vi "开机添加默认配置文件.vi"(8 "error in (no error)":errorcluster caption="错误输入（无错误）", 11 "恢复默认方式":enum16{"无配置开机恢复", "手动恢复"}(ring)) -> (0 "error out":errorcluster caption="错误输出")   [LabVIEW 2016, in "环境动力监测库.lvlib"]
uses:
  <vilib>/Utility/config.llb/NI_LVConfig.lvlib
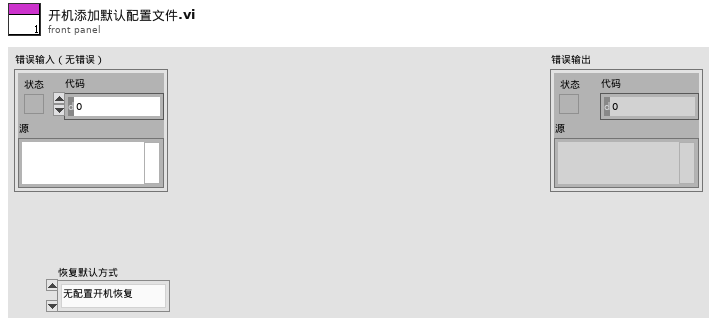
[diagram p1: front panel]
types:
  T1 = cluster{"监测项描述:输出":string, "端口":enum16{"AI0", "AI1", "AI2", "AI3", "AI4", "DI0", "DI1", "DI2", "DI3", "DI4", "DI5", "DI6", "DI7", "DO0", "DO1", "DO2", "DO3", "DO4", "DO5", "DO6", "DO7", "X0", "X1", "X2", "X3", "X4", "X5", "X6", "X7", "X8", "X9", "X10", "X11", "X12", "X13", "X14", "X15", "X16", "X17", "X18", "X19", "X20", "X21", "X22", "X23"}, "告警方式":enum32{"禁用告警", "闭合告警", "断开告警"}, "传感器型号":enum16{"PLC", "ZLAN", "ART"}, "声光告警启用":bool}
  T2 = typedef "NI_LVConfig.lvlib/Config Data RefNum.ctl" = refnum<k1>
  T3 = cluster{"监测项描述:输出":string, "连接方式":enum16{"串口", "TCP"}, "端口":string, "IP address:":string, "Port:":string, "站号":u64, "传感器型号":string, "波特率":u64, "data bits":u64, "停止位":u16, "奇偶校验":u16}
  T4 = cluster{"监测项描述:输出":string, "端口":enum16{"AI0", "AI1", "AI2", "AI3", "AI4", "DI0", "DI1", "DI2", "DI3", "DI4", "DO0", "DO1", "DO2", "DO3", "DO4", "X0", "X1", "X2", "X3", "X4", "X5", "X6", "X7", "X8", "X9"}, "告警方式":enum32{"禁用告警", "闭合告警", "断开告警"}, "传感器型号":enum16{"PLC", "ZLAN"}}
  T5 = enum16{"AI0", "AI1", "AI2", "AI3", "AI4", "DI0", "DI1", "DI2", "DI3", "DI4", "DI5", "DI6", "DI7", "DO0", "DO1", "DO2", "DO3", "DO4", "DO5", "DO6", "DO7", "X0", "X1", "X2", "X3", "X4", "X5", "X6", "X7", "X8", "X9"}[]
  T6 = cluster{"漏水监测配置":cluster{"监测项描述:输出":string, "端口:":enum16{"AI0", "AI1", "AI2", "AI3", "AI4", "DI0", "DI1", "DI2", "DI3", "DI4", "DI5", "DI6", "DI7", "DO0", "DO1", "DO2", "DO3", "DO4", "DO5", "DO6", "DO7", "X0", "X1", "X2", "X3", "X4", "X5", "X6", "X7", "X8", "X9", "X10", "X11", "X12", "X13", "X14", "X15", "X16", "X17", "X18", "X19", "X20", "X21", "X22", "X23"}, "告警参数:":enum32{"禁用告警", "闭合告警", "断开告警"}, "传感器型号:":enum16{"PLC", "ZLAN", "ART"}, "声光告警启用":bool}, "门禁开关监测配置":cluster{"监测项描述:输出":string, "端口:":enum16{"AI0", "AI1", "AI2", "AI3", "AI4", "DI0", "DI1", "DI2", "DI3", "DI4", "DI5", "DI6", "DI7", "DO0", "DO1", "DO2", "DO3", "DO4", "DO5", "DO6", "DO7", "X0", "X1", "X2", "X3", "X4", "X5", "X6", "X7", "X8", "X9", "X10", "X11", "X12", "X13", "X14", "X15", "X16", "X17", "X18", "X19", "X20", "X21", "X22", "X23"}, "告警参数:":enum32{"禁用告警", "闭合告警", "断开告警"}, "传感器型号:":enum16{"PLC", "ZLAN", "ART"}, "声光告警启用":bool}, "门禁开关监测配置2":cluster{"监测项描述:输出":string, "端口:":enum16{"AI0", "AI1", "AI2", "AI3", "AI4", "DI0", "DI1", "DI2", "DI3", "DI4", "DI5", "DI6", "DI7", "DO0", "DO1", "DO2", "DO3", "DO4", "DO5", "DO6", "DO7", "X0", "X1", "X2", "X3", "X4", "X5", "X6", "X7", "X8", "X9", "X10", "X11", "X12", "X13", "X14", "X15", "X16", "X17", "X18", "X19", "X20", "X21", "X22", "X23"}, "告警参数:":enum32{"禁用告警", "闭合告警", "断开告警"}, "传感器型号:":enum16{"PLC", "ZLAN", "ART"}, "声光告警启用":bool}, "温湿度监测配置":cluster{"监测项描述:输出":string, "端口:":enum16{"AI0", "AI1", "AI2", "AI3", "AI4", "DI0", "DI1", "DI2", "DI3", "DI4", "DI5", "DI6", "DI7", "DO0", "DO1", "DO2", "DO3", "DO4", "DO5", "DO6", "DO7", "X0", "X1", "X2", "X3", "X4", "X5", "X6", "X7", "X8", "X9", "X10", "X11", "X12", "X13", "X14", "X15", "X16", "X17", "X18", "X19", "X20", "X21", "X22", "X23"}, "告警参数:":enum32{"禁用告警", "闭合告警", "断开告警"}, "传感器型号:":enum16{"PLC", "ZLAN", "ART"}, "声光告警启用":bool}, "烟雾监测配置":cluster{"监测项描述:输出":string, "端口:":enum16{"AI0", "AI1", "AI2", "AI3", "AI4", "DI0", "DI1", "DI2", "DI3", "DI4", "DI5", "DI6", "DI7", "DO0", "DO1", "DO2", "DO3", "DO4", "DO5", "DO6", "DO7", "X0", "X1", "X2", "X3", "X4", "X5", "X6", "X7", "X8", "X9", "X10", "X11", "X12", "X13", "X14", "X15", "X16", "X17", "X18", "X19", "X20", "X21", "X22", "X23"}, "告警参数:":enum32{"禁用告警", "闭合告警", "断开告警"}, "传感器型号:":enum16{"PLC", "ZLAN", "ART"}, "声光告警启用":bool}, "冰箱监测配置":cluster{"监测项描述:输出":string, "端口:":enum16{"AI0", "AI1", "AI2", "AI3", "AI4", "DI0", "DI1", "DI2", "DI3", "DI4", "DI5", "DI6", "DI7", "DO0", "DO1", "DO2", "DO3", "DO4", "DO5", "DO6", "DO7", "X0", "X1", "X2", "X3", "X4", "X5", "X6", "X7", "X8", "X9", "X10", "X11", "X12", "X13", "X14", "X15", "X16", "X17", "X18", "X19", "X20", "X21", "X22", "X23"}, "告警参数:":enum32{"禁用告警", "闭合告警", "断开告警"}, "传感器型号:":enum16{"PLC", "ZLAN", "ART"}, "声光告警启用":bool}, "排气扇监测配置":cluster{"监测项描述:输出":string, "端口:":enum16{"AI0", "AI1", "AI2", "AI3", "AI4", "DI0", "DI1", "DI2", "DI3", "DI4", "DI5", "DI6", "DI7", "DO0", "DO1", "DO2", "DO3", "DO4", "DO5", "DO6", "DO7", "X0", "X1", "X2", "X3", "X4", "X5", "X6", "X7", "X8", "X9", "X10", "X11", "X12", "X13", "X14", "X15", "X16", "X17", "X18", "X19", "X20", "X21", "X22", "X23"}, "告警参数:":enum32{"禁用告警", "闭合告警", "断开告警"}, "传感器型号:":enum16{"PLC", "ZLAN", "ART"}, "声光告警启用":bool}, "红外入侵监测配置":cluster{"监测项描述:输出":string, "端口:":enum16{"AI0", "AI1", "AI2", "AI3", "AI4", "DI0", "DI1", "DI2", "DI3", "DI4", "DI5", "DI6", "DI7", "DO0", "DO1", "DO2", "DO3", "DO4", "DO5", "DO6", "DO7", "X0", "X1", "X2", "X3", "X4", "X5", "X6", "X7", "X8", "X9", "X10", "X11", "X12", "X13", "X14", "X15", "X16", "X17", "X18", "X19", "X20", "X21", "X22", "X23"}, "告警参数:":enum32{"禁用告警", "闭合告警", "断开告警"}, "传感器型号:":enum16{"PLC", "ZLAN", "ART"}, "声光告警启用":bool}, "振动监测配置":cluster{"监测项描述:输出":string, "端口:":enum16{"AI0", "AI1", "AI2", "AI3", "AI4", "DI0", "DI1", "DI2", "DI3", "DI4", "DI5", "DI6", "DI7", "DO0", "DO1", "DO2", "DO3", "DO4", "DO5", "DO6", "DO7", "X0", "X1", "X2", "X3", "X4", "X5", "X6", "X7", "X8", "X9", "X10", "X11", "X12", "X13", "X14", "X15", "X16", "X17", "X18", "X19", "X20", "X21", "X22", "X23"}, "告警参数:":enum32{"禁用告警", "闭合告警", "断开告警"}, "传感器型号:":enum16{"PLC", "ZLAN", "ART"}, "声光告警启用":bool}, "废液监测配置":cluster{"监测项描述:输出":string, "端口:":enum16{"AI0", "AI1", "AI2", "AI3", "AI4", "DI0", "DI1", "DI2", "DI3", "DI4", "DI5", "DI6", "DI7", "DO0", "DO1", "DO2", "DO3", "DO4", "DO5", "DO6", "DO7", "X0", "X1", "X2", "X3", "X4", "X5", "X6", "X7", "X8", "X9", "X10", "X11", "X12", "X13", "X14", "X15", "X16", "X17", "X18", "X19", "X20", "X21", "X22", "X23"}, "告警参数:":enum32{"禁用告警", "闭合告警", "断开告警"}, "传感器型号:":enum16{"PLC", "ZLAN", "ART"}, "声光告警启用":bool}, "废液监测配置2":cluster{"监测项描述:输出":string, "端口:":enum16{"AI0", "AI1", "AI2", "AI3", "AI4", "DI0", "DI1", "DI2", "DI3", "DI4", "DI5", "DI6", "DI7", "DO0", "DO1", "DO2", "DO3", "DO4", "DO5", "DO6", "DO7", "X0", "X1", "X2", "X3", "X4", "X5", "X6", "X7", "X8", "X9", "X10", "X11", "X12", "X13", "X14", "X15", "X16", "X17", "X18", "X19", "X20", "X21", "X22", "X23"}, "告警参数:":enum32{"禁用告警", "闭合告警", "断开告警"}, "传感器型号:":enum16{"PLC", "ZLAN", "ART"}, "声光告警启用":bool}}
  T7 = cluster{"市电监测":bool, "用水量监测":bool, "烟雾监测":bool, "温度湿度":bool, "振动监测":bool, "红外入侵监测":bool, "漏水监测":bool, "门禁开关监测":bool, "门禁开关监测2":bool, "视频监测":bool, "UPS监测":bool, "空调监测":bool, "冰箱监测":bool, "排气扇监测":bool, "蓄电池监测":bool, "蓄电池监测2":bool, "GPS监测":bool, "北斗监测":bool, "气象监测":bool, "智能门禁监测":bool, "废液监测":bool, "废液监测2":bool}
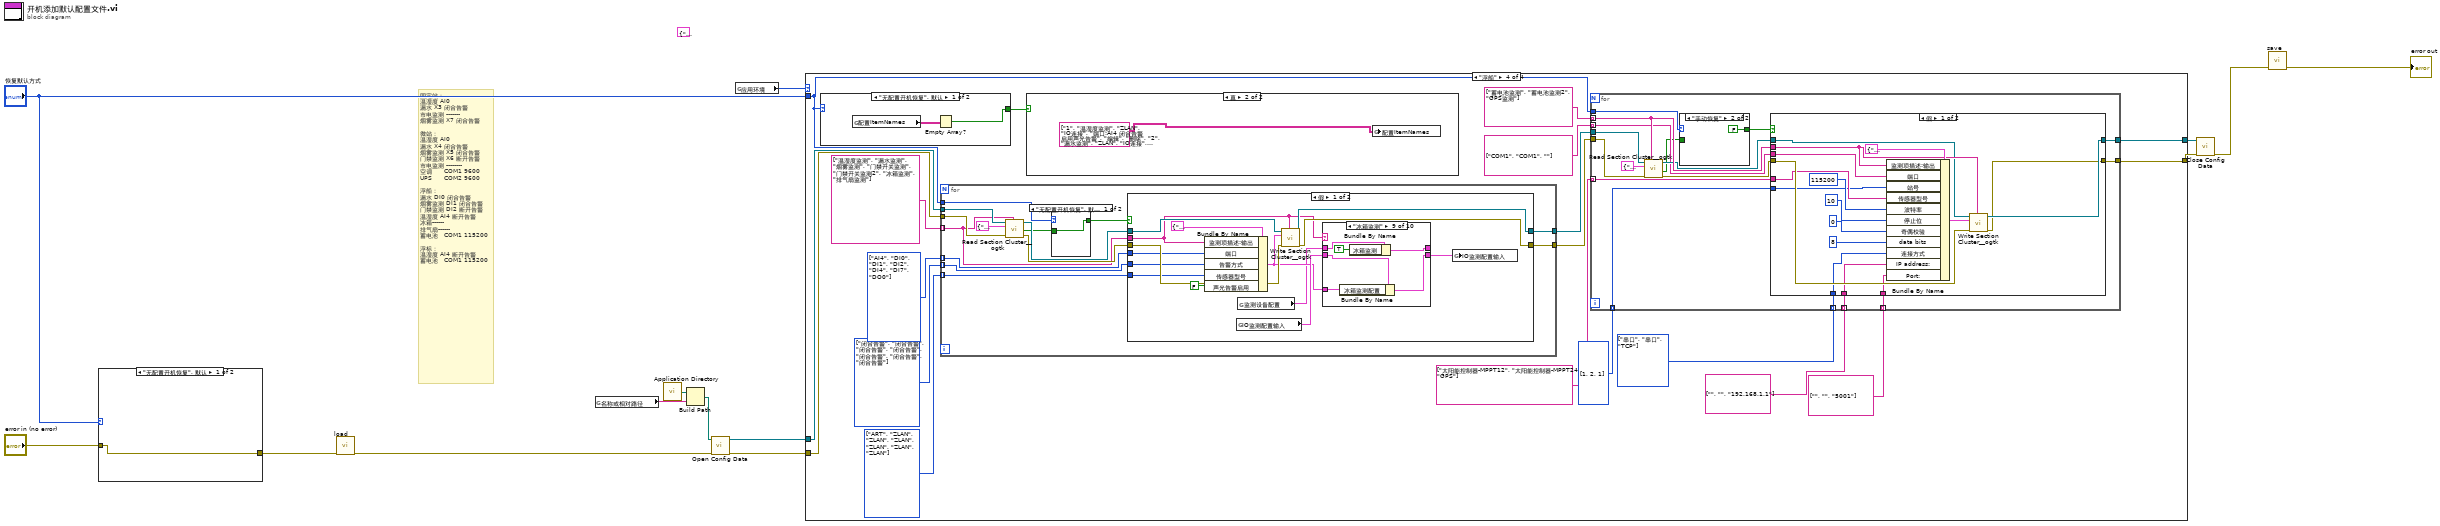
[diagram p0: block diagram]
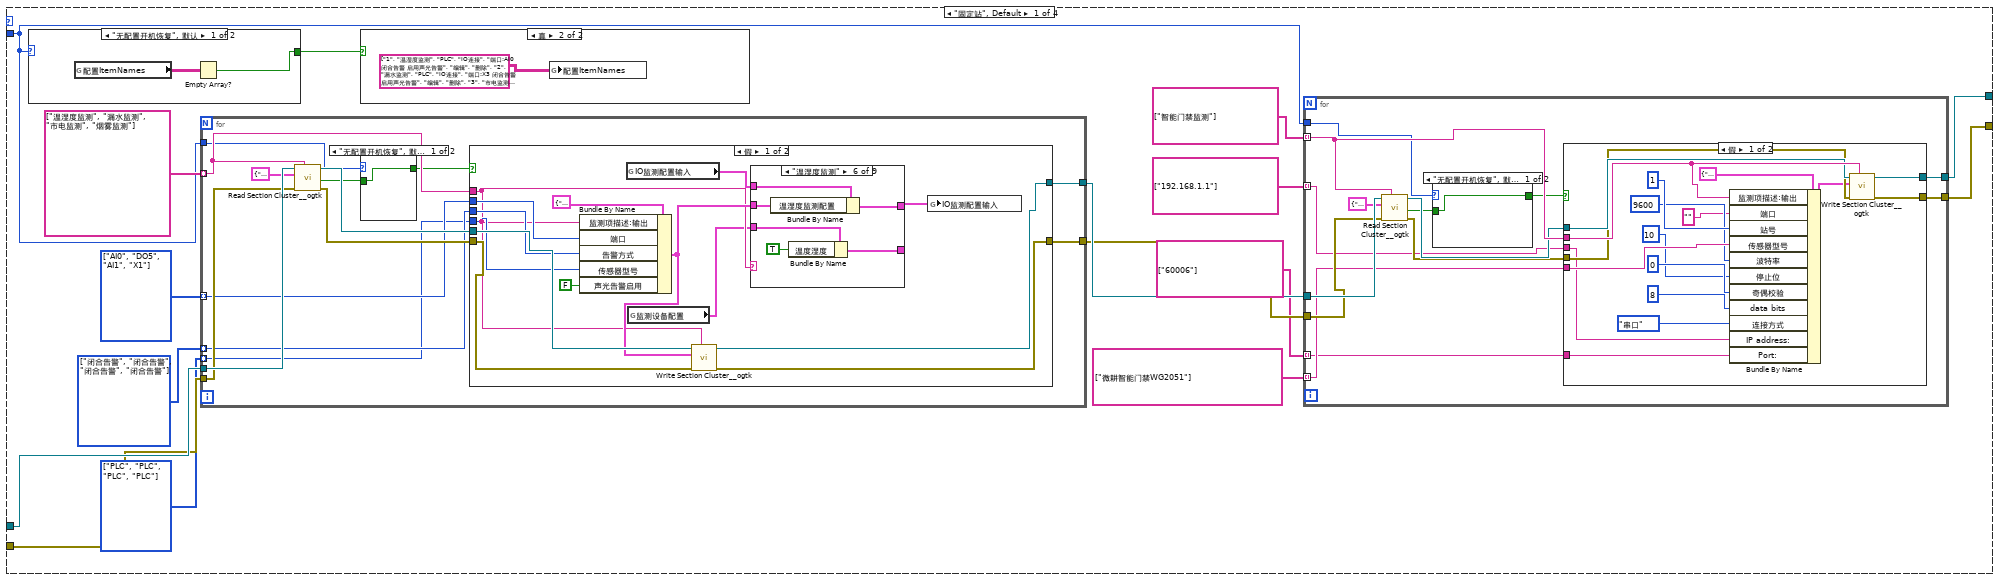
[diagram p3: hidden frame]
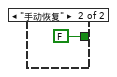
[diagram p4: hidden frame]
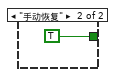
[diagram p6: hidden frame]
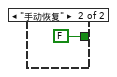
[diagram p8: hidden frame]
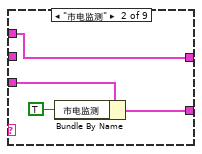
[diagram p10: hidden frame]
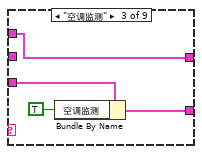
[diagram p11: hidden frame]
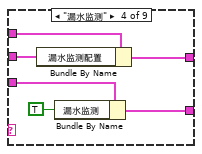
[diagram p12: hidden frame]
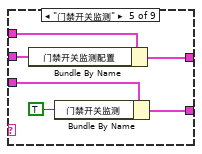
[diagram p13: hidden frame]
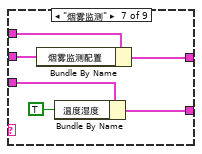
[diagram p14: hidden frame]
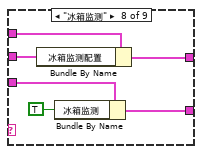
[diagram p15: hidden frame]
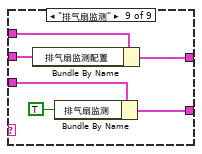
[diagram p16: hidden frame]
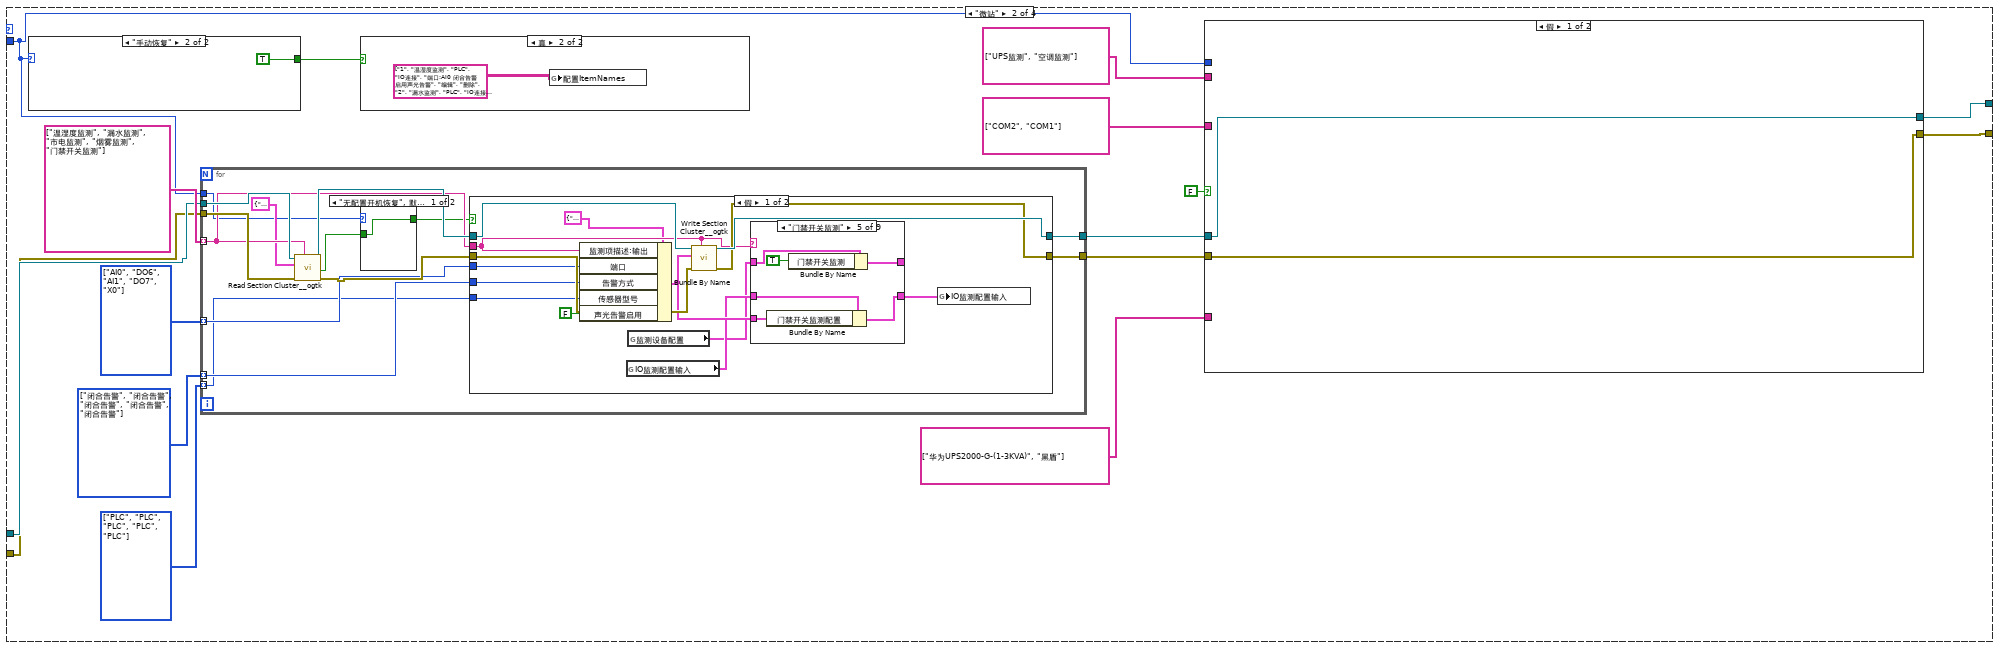
[diagram p18: hidden frame]
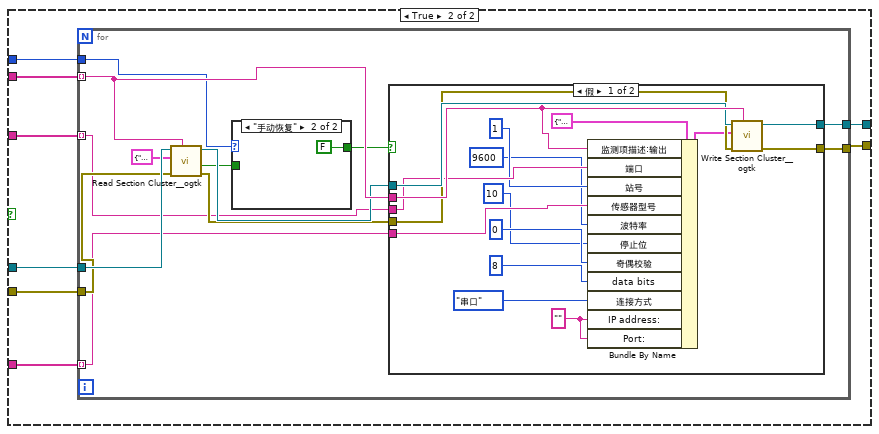
[diagram p19: hidden frame]
diagram:
  (unwired) T1 {"监测项描述:输出"="", "端口"=enum."AI0", "告警方式"=enum."禁用告警", "传感器型号"=enum."PLC", "声光告警启用"=FALSE} ("簇1输入")
  # "固定站：\n温湿度 AI0\n漏水 X3 闭合告警\n市电监测 -------\n烟雾监测 X7 闭合告警\n\n微站：\n温湿度 AI0\n漏水 X4 闭合告警\n烟雾监测 X5 闭合告警\n门禁监测 X6 断开告警\n市电监测 --------\n空调      COM1 9600\nUPS      COM2 9600\n\n浮船：\n漏水 DI0 闭合告警\n烟雾监测 DI1 闭合告警\n门禁监测 DI2 断开告警\n温湿度 AI4 断开告警\n冰箱------\n排气扇------\n蓄电池   COM1 115200\n\n浮标：\n温湿度 AI4 断开告警\n蓄电池   COM1 115200"
  n1 = case shown="\"无配置开机恢复\", 默认" "恢复默认方式" {
    tunnel: "error in (no error)" -> [w15 w16]
    tunnel: [w15 w16] -> w3
    frame "无配置开机恢复", Default {
    }
    frame "手动恢复" {
    }
  }
  n2 = call "load.vi"("error in (no error)"=w3) -> ("error out"=w7:errorcluster)  [unwired: 10 in]
  n3 = global read "内部交互全局变量.vi" "名称或相对路径"() -> (w4:string)
  n4 = call <vilib>:"Application Directory.vi"() -> ("Application Directory"=w13:path)
  n5 = Build Path(base path=w13, name or relative path=w4) -> (appended path=w12:path)
  n6 = call <vilib>:"Open Config Data.vi"("error in (no error)"=w7, "configuration file path"=w12) -> ("error out"=w10:errorcluster, "refnum"=w11:T2)  [unwired: 7 in, 1 out]
  n7 = global read "外部交互全局变量.vi" "应用环境"() -> (w14:enum16{"固定站", "微站", "浮标", "浮船"})
  n8 = case shown="\"浮船\"" w14 {
    tunnel: w11 -> [w31 w164 w304 w438]
    tunnel: w10 -> [w30 w163 w303 w437]
    tunnel: [w19 w159 w299 w433] -> w9
    tunnel: [w18 w158 w298 w432] -> w8
    tunnel: "恢复默认方式" -> [w20 w151 w291 w425]
    frame "固定站", Default {
      w27 = enum16{"PLC", "ZLAN"}[] [enum."PLC", enum."PLC", enum."PLC", enum."PLC"] items=["PLC", "ZLAN"]
      w28 = enum32{"禁用告警", "闭合告警", "断开告警"}[] [enum."闭合告警", enum."闭合告警", enum."闭合告警", enum."闭合告警"] items=["禁用告警", "闭合告警", "断开告警"]
      w29 = T5 [enum."AI0", enum."DO5", enum."AI1", enum."X1"] items=["AI0", "AI1", "AI2", "AI3", "AI4", "DI0", "DI1", "DI2", "DI3", "DI4", "DI5", "DI6", "DI7", "DO0", "DO1", "DO2", "DO3", "DO4", "DO5", "DO6", "DO7", "X0", "X1", "X2", "X3", "X4", "X5", "X6", "X7", "X8", "X9"]
      n9 = case shown="\"无配置开机恢复\", 默认" w20 {
        tunnel: [w68 TRUE ("empty?")] -> w26
        frame "无配置开机恢复", Default {
          n10 = global read "断电保存全局变量.vi" "配置ItemNames"() -> (w69:string[][])
          n11 = Empty Array?(array=w69) -> (empty?=w68:bool)
        }
        frame "手动恢复" {
        }
      }
      n12 = for {
        tunnel: string[] ["温湿度监测", "漏水监测", "市电监测", "烟雾监测"] -> [w81] mode=indexing
        tunnel: w31 -> [w85]
        tunnel: w30 -> [w84]
        tunnel: w29 -> [w80] mode=indexing
        tunnel: w28 -> [w79] mode=indexing
        tunnel: w27 -> [w78] mode=indexing
        tunnel: [w77] -> w22
        tunnel: [w76] -> w21
        tunnel: w20 -> [w72]
        n13 = call <userlib>:"Read Section Cluster__ogtk.vi"("section (optional)"=w81, "error in (no error)"=w84, "Section Formatted Cluster Type"=T4 {"监测项描述:输出"="烟雾监测", "端口"=enum."X8", "告警方式"=enum."闭合告警", "传感器型号"=enum."PLC"} ("簇1输入"), "refnum"=w85) -> ("error out"=w82:errorcluster, "all found?"=w74:bool, "dup refnum"=w83:T2)  [unwired: 3 in, 2 out]
        n14 = case shown="\"无配置开机恢复\", 默认" w72 {
          tunnel: [w86 FALSE] -> w73
          tunnel: w74 -> [w86 _]
          frame "无配置开机恢复", Default {
          }
          frame "手动恢复" {
          }
        }
        n15 = case shown="假" w73 {
          tunnel: w83 -> [w101 w149]
          tunnel: w82 -> [w100 w148]
          tunnel: w81 -> [w92 _]
          tunnel: w80 -> [w99 _]
          tunnel: w79 -> [w94 _]
          tunnel: w78 -> [w98 _]
          tunnel: [w97 w149] -> w77
          tunnel: [w96 w148] -> w76
          frame False {
            n16 = Bundle By Name(cluster=T1 {"监测项描述:输出"="", "端口"=enum."AI0", "告警方式"=enum."禁用告警", "传感器型号"=enum."PLC", "声光告警启用"=FALSE} ("簇1输入"), "监测项描述:输出"=w92, "端口"=w99, "告警方式"=w94, "传感器型号"=w98, "声光告警启用"=FALSE) -> (w93:T1)
            n17 = global read "断电保存全局变量.vi" "IO监测配置输入"() -> (w95:T6)
            n18 = global read "断电保存全局变量.vi" "监测设备配置"() -> (w91:T7)
            n19 = call <userlib>:"Write Section Cluster__ogtk.vi"("section (optional)"=w92, "error in (no error)"=w100, "Section Formatted Cluster"=w93, "refnum"=w101) -> ("error out"=w96:errorcluster, "dup refnum"=w97:T2)  [unwired: 6 in]
            n20 = case shown="\"温湿度监测\"" w92 {
              tunnel: w95 -> [w103 w107 w111 w117 w123 w129 w135 w141 w147]
              tunnel: [w103 w107 w111 w116 w122 w128 w134 w140 w146] -> w90
              tunnel: w93 -> [_ _ _ w115 w121 w127 w133 w139 w145]
              tunnel: w91 -> [w102 w106 w110 w114 w119 w126 w132 w138 w144]
              tunnel: [w102 w104 w109 w113 w120 w125 w131 w137 w143] -> _
              frame "假", Default {
              }
              frame "市电监测" {
                n21 = Bundle By Name(cluster=w106, "市电监测"=TRUE) -> (w104:T7)
              }
              frame "空调监测" {
                n22 = Bundle By Name(cluster=w110, "空调监测"=TRUE) -> (w109:T7)
              }
              frame "漏水监测" {
                n23 = Bundle By Name(cluster=w117, "漏水监测配置"=w115) -> (w116:T6)
                n24 = Bundle By Name(cluster=w114, "漏水监测"=TRUE) -> (w113:T7)
              }
              frame "门禁开关监测" {
                n25 = Bundle By Name(cluster=w123, "门禁开关监测配置"=w121) -> (w122:T6)
                n26 = Bundle By Name(cluster=w119, "门禁开关监测"=TRUE) -> (w120:T7)
              }
              frame "温湿度监测" {
                n27 = Bundle By Name(cluster=w129, "温湿度监测配置"=w127) -> (w128:T6)
                n28 = Bundle By Name(cluster=w126, "温度湿度"=TRUE) -> (w125:T7)
              }
              frame "烟雾监测" {
                n29 = Bundle By Name(cluster=w135, "烟雾监测配置"=w133) -> (w134:T6)
                n30 = Bundle By Name(cluster=w132, "温度湿度"=TRUE) -> (w131:T7)
              }
              frame "冰箱监测" {
                n31 = Bundle By Name(cluster=w141, "冰箱监测配置"=w139) -> (w140:T6)
                n32 = Bundle By Name(cluster=w138, "冰箱监测"=TRUE ("市电监测")) -> (w137:T7)
              }
              frame "排气扇监测" {
                n33 = Bundle By Name(cluster=w147, "排气扇监测配置"=w145) -> (w146:T6)
                n34 = Bundle By Name(cluster=w144, "排气扇监测"=TRUE) -> (w143:T7)
              }
            }
            n35 = global write "断电保存全局变量.vi" "IO监测配置输入"(w90) -> ()
          }
          frame True {
          }
        }
      }
      n36 = case shown="真" w26 {
        frame False {
        }
        frame True {
          n37 = global write "断电保存全局变量.vi" "配置ItemNames"(string[][] [["1", "温湿度监测", "PLC", "IO连接", "端口:AI0 闭合告警 启用声光告警", "编辑", "删除"], ["2", "漏水监测", "PLC", "IO连接", "端口:X3 闭合告警 启用声光告警", "编辑", "删除"], ["3", "市电监测", "PLC", "IO连接", "端口:AI1 闭合告警 启用声光告警", "编辑", "删除"], ["4", "烟雾监测", "PLC", "IO连接", "端口:X7 闭合告警 启用声光告警", "编辑", "删除"], ["5", "智能门禁监测", "微耕智能门禁WG2051", "TCP连接", "IP:127.0.0.1 Port:60006 不启用声光告警", "编辑", "删除"]] ("配置ItemNames")) -> ()
        }
      }
      n38 = for {
        tunnel: w22 -> [w46]
        tunnel: w21 -> [w45]
        tunnel: string[] ["智能门禁监测"] -> [w44] mode=indexing
        tunnel: [w41] -> w19
        tunnel: [w40] -> w18
        tunnel: string[] ["192.168.1.1"] -> [w39] mode=indexing
        tunnel: string[] ["微耕智能门禁WG2051"] -> [w38] mode=indexing
        tunnel: w20 -> [w36]
        tunnel: string[] ["60006"] -> [w33] mode=indexing
        n39 = call <userlib>:"Read Section Cluster__ogtk.vi"("section (optional)"=w44, "error in (no error)"=w45, "Section Formatted Cluster Type"=T3 {"监测项描述:输出"="", "连接方式"=enum."串口", "端口"="", "IP address:"="", "Port:"="", "站号"=19200, "传感器型号"="", "波特率"=19200, "data bits"=8, "停止位"=10, "奇偶校验"=0} ("输出簇"), "refnum"=w46) -> ("error out"=w42:errorcluster, "all found?"=w35:bool, "dup refnum"=w43:T2)  [unwired: 3 in, 2 out]
        n40 = case shown="\"无配置开机恢复\", 默认" w36 {
          tunnel: [w47 FALSE] -> w34
          tunnel: w35 -> [w47 _]
          frame "无配置开机恢复", Default {
          }
          frame "手动恢复" {
          }
        }
        n41 = case shown="假" w34 {
          tunnel: w44 -> [w64 _]
          tunnel: w43 -> [w63 w67]
          tunnel: w42 -> [w62 w66]
          tunnel: [w60 w67] -> w41
          tunnel: [w59 w66] -> w40
          tunnel: w39 -> [w50 _]
          tunnel: w38 -> [w57 _]
          tunnel: w33 -> [w49 _]
          frame False {
            n42 = Bundle By Name(cluster=T3 {"监测项描述:输出"="", "连接方式"=enum."串口", "端口"="", "IP address:"="", "Port:"="", "站号"=19200, "传感器型号"="", "波特率"=19200, "data bits"=8, "停止位"=10, "奇偶校验"=0} ("输出簇"), "监测项描述:输出"=w64, "端口"="" ("IP address:"), "站号"=u64 1, "传感器型号"=w57, "波特率"=u64 9600, "停止位"=u16 10, "奇偶校验"=u16 0, "data bits"=u64 8, "连接方式"=enum16{"串口", "TCP"}."串口", "IP address:"=w50, "Port:"=w49) -> (w61:T3)
            n43 = call <userlib>:"Write Section Cluster__ogtk.vi"("section (optional)"=w64, "error in (no error)"=w62, "Section Formatted Cluster"=w61, "refnum"=w63) -> ("error out"=w59:errorcluster, "dup refnum"=w60:T2)  [unwired: 6 in]
          }
          frame True {
          }
        }
      }
    }
    frame "微站" {
      w153 = enum16{"PLC", "ZLAN"}[] [enum."PLC", enum."PLC", enum."PLC", enum."PLC", enum."PLC"] items=["PLC", "ZLAN"]
      w154 = enum32{"禁用告警", "闭合告警", "断开告警"}[] [enum."闭合告警", enum."闭合告警", enum."闭合告警", enum."闭合告警", enum."闭合告警"] items=["禁用告警", "闭合告警", "断开告警"]
      w155 = T5 [enum."AI0", enum."DO6", enum."AI1", enum."DO7", enum."X0"] items=["AI0", "AI1", "AI2", "AI3", "AI4", "DI0", "DI1", "DI2", "DI3", "DI4", "DI5", "DI6", "DI7", "DO0", "DO1", "DO2", "DO3", "DO4", "DO5", "DO6", "DO7", "X0", "X1", "X2", "X3", "X4", "X5", "X6", "X7", "X8", "X9"]
      n44 = case shown="\"手动恢复\"" w151 {
        tunnel: [w209 TRUE ("empty?")] -> w152
        frame "无配置开机恢复", Default {
          n45 = global read "断电保存全局变量.vi" "配置ItemNames"() -> (w210:string[][])
          n46 = Empty Array?(array=w210) -> (empty?=w209:bool)
        }
        frame "手动恢复" {
        }
      }
      n47 = for {
        tunnel: string[] ["温湿度监测", "漏水监测", "市电监测", "烟雾监测", "门禁开关监测"] -> [w222] mode=indexing
        tunnel: w164 -> [w226]
        tunnel: w163 -> [w225]
        tunnel: w155 -> [w221] mode=indexing
        tunnel: w154 -> [w220] mode=indexing
        tunnel: w153 -> [w219] mode=indexing
        tunnel: [w218] -> w162
        tunnel: [w217] -> w161
        tunnel: w151 -> [w215]
        n48 = call <userlib>:"Read Section Cluster__ogtk.vi"("section (optional)"=w222, "error in (no error)"=w225, "Section Formatted Cluster Type"=T4 {"监测项描述:输出"="烟雾监测", "端口"=enum."X8", "告警方式"=enum."闭合告警", "传感器型号"=enum."PLC"} ("簇1输入"), "refnum"=w226) -> ("error out"=w223:errorcluster, "all found?"=w214:bool, "dup refnum"=w224:T2)  [unwired: 3 in, 2 out]
        n49 = case shown="\"无配置开机恢复\", 默认" w215 {
          tunnel: [w227 FALSE] -> w213
          tunnel: w214 -> [w227 _]
          frame "无配置开机恢复", Default {
          }
          frame "手动恢复" {
          }
        }
        n50 = case shown="假" w213 {
          tunnel: w224 -> [w242 w290]
          tunnel: w223 -> [w241 w289]
          tunnel: w222 -> [w235 _]
          tunnel: w221 -> [w240 _]
          tunnel: w220 -> [w239 _]
          tunnel: w219 -> [w238 _]
          tunnel: [w237 w290] -> w218
          tunnel: [w236 w289] -> w217
          frame False {
            n51 = Bundle By Name(cluster=T1 {"监测项描述:输出"="", "端口"=enum."AI0", "告警方式"=enum."禁用告警", "传感器型号"=enum."PLC", "声光告警启用"=FALSE} ("簇1输入"), "监测项描述:输出"=w235, "端口"=w240, "告警方式"=w239, "传感器型号"=w238, "声光告警启用"=FALSE) -> (w234:T1)
            n52 = global read "断电保存全局变量.vi" "IO监测配置输入"() -> (w233:T6)
            n53 = global read "断电保存全局变量.vi" "监测设备配置"() -> (w231:T7)
            n54 = call <userlib>:"Write Section Cluster__ogtk.vi"("section (optional)"=w235, "error in (no error)"=w241, "Section Formatted Cluster"=w234, "refnum"=w242) -> ("error out"=w236:errorcluster, "dup refnum"=w237:T2)  [unwired: 6 in]
            n55 = case shown="\"门禁开关监测\"" w235 {
              tunnel: w233 -> [w244 w248 w252 w258 w264 w270 w276 w282 w288]
              tunnel: [w244 w248 w252 w257 w263 w269 w275 w281 w287] -> w232
              tunnel: w234 -> [_ _ _ w256 w262 w268 w274 w280 w286]
              tunnel: w231 -> [w243 w247 w251 w255 w260 w267 w273 w279 w285]
              tunnel: [w243 w245 w250 w254 w261 w266 w272 w278 w284] -> _
              frame "假", Default {
              }
              frame "市电监测" {
                n56 = Bundle By Name(cluster=w247, "市电监测"=TRUE) -> (w245:T7)
              }
              frame "空调监测" {
                n57 = Bundle By Name(cluster=w251, "空调监测"=TRUE) -> (w250:T7)
              }
              frame "漏水监测" {
                n58 = Bundle By Name(cluster=w258, "漏水监测配置"=w256) -> (w257:T6)
                n59 = Bundle By Name(cluster=w255, "漏水监测"=TRUE) -> (w254:T7)
              }
              frame "门禁开关监测" {
                n60 = Bundle By Name(cluster=w264, "门禁开关监测配置"=w262) -> (w263:T6)
                n61 = Bundle By Name(cluster=w260, "门禁开关监测"=TRUE) -> (w261:T7)
              }
              frame "温湿度监测" {
                n62 = Bundle By Name(cluster=w270, "温湿度监测配置"=w268) -> (w269:T6)
                n63 = Bundle By Name(cluster=w267, "温度湿度"=TRUE) -> (w266:T7)
              }
              frame "烟雾监测" {
                n64 = Bundle By Name(cluster=w276, "烟雾监测配置"=w274) -> (w275:T6)
                n65 = Bundle By Name(cluster=w273, "温度湿度"=TRUE) -> (w272:T7)
              }
              frame "冰箱监测" {
                n66 = Bundle By Name(cluster=w282, "冰箱监测配置"=w280) -> (w281:T6)
                n67 = Bundle By Name(cluster=w279, "冰箱监测"=TRUE ("市电监测")) -> (w278:T7)
              }
              frame "排气扇监测" {
                n68 = Bundle By Name(cluster=w288, "排气扇监测配置"=w286) -> (w287:T6)
                n69 = Bundle By Name(cluster=w285, "排气扇监测"=TRUE) -> (w284:T7)
              }
            }
            n70 = global write "断电保存全局变量.vi" "IO监测配置输入"(w232) -> ()
          }
          frame True {
          }
        }
      }
      n71 = case shown="真" w152 {
        frame False {
        }
        frame True {
          n72 = global write "断电保存全局变量.vi" "配置ItemNames"(string[][] [["1", "温湿度监测", "PLC", "IO连接", "端口:AI0 闭合告警 启用声光告警", "编辑", "删除"], ["2", "漏水监测", "PLC", "IO连接", "端口:X4 闭合告警 启用声光告警", "编辑", "删除"], ["3", "市电监测", "PLC", "IO连接", "端口:AI1 闭合告警 启用声光告警", "编辑", "删除"], ["4", "烟雾监测", "PLC", "IO连接", "端口:X5 闭合告警 启用声光告警", "编辑", "删除"], ["5", "门禁开关监测", "PLC", "IO连接", "端口:X6 闭合告警 启用声光告警", "编辑", "删除"]] ("配置ItemNames")) -> ()
        }
      }
      n73 = case shown="假" FALSE {
        tunnel: w162 -> [w167 w175]
        tunnel: w161 -> [w166 w174]
        tunnel: string[] ["UPS监测", "空调监测"] -> [_ w173]
        tunnel: [w167 w172] -> w159
        tunnel: [w166 w171] -> w158
        tunnel: string[] ["COM2", "COM1"] -> [_ w170]
        tunnel: string[] ["华为UPS2000-G-(1-3KVA)", "黑盾"] -> [_ w169]
        tunnel: w151 -> [_ w168]
        frame False {
        }
        frame True {
          n74 = for {
            tunnel: w175 -> [w188]
            tunnel: w174 -> [w187]
            tunnel: w173 -> [w186] mode=indexing
            tunnel: [w183] -> w172
            tunnel: [w182] -> w171
            tunnel: w170 -> [w181] mode=indexing
            tunnel: w169 -> [w180] mode=indexing
            tunnel: w168 -> [w178]
            n75 = call <userlib>:"Read Section Cluster__ogtk.vi"("section (optional)"=w186, "error in (no error)"=w187, "Section Formatted Cluster Type"=T3 {"监测项描述:输出"="", "连接方式"=enum."串口", "端口"="", "IP address:"="", "Port:"="", "站号"=19200, "传感器型号"="", "波特率"=19200, "data bits"=8, "停止位"=10, "奇偶校验"=0} ("输出簇"), "refnum"=w188) -> ("error out"=w184:errorcluster, "all found?"=w177:bool, "dup refnum"=w185:T2)  [unwired: 3 in, 2 out]
            n76 = case shown="\"手动恢复\"" w178 {
              tunnel: [w189 FALSE] -> w176
              tunnel: w177 -> [w189 _]
              frame "无配置开机恢复", Default {
              }
              frame "手动恢复" {
              }
            }
            n77 = case shown="假" w176 {
              tunnel: w186 -> [w205 _]
              tunnel: w185 -> [w204 w208]
              tunnel: w184 -> [w203 w207]
              tunnel: [w201 w208] -> w183
              tunnel: [w200 w207] -> w182
              tunnel: w181 -> [w199 _]
              tunnel: w180 -> [w197 _]
              frame False {
                w191 = "" ("IP address:")
                n78 = Bundle By Name(cluster=T3 {"监测项描述:输出"="", "连接方式"=enum."串口", "端口"="", "IP address:"="", "Port:"="", "站号"=19200, "传感器型号"="", "波特率"=19200, "data bits"=8, "停止位"=10, "奇偶校验"=0} ("输出簇"), "监测项描述:输出"=w205, "端口"=w199, "站号"=u64 1, "传感器型号"=w197, "波特率"=u64 9600, "停止位"=u16 10, "奇偶校验"=u16 0, "data bits"=u64 8, "连接方式"=enum16{"串口", "TCP"}."串口", "IP address:"=w191, "Port:"=w191) -> (w202:T3)
                n79 = call <userlib>:"Write Section Cluster__ogtk.vi"("section (optional)"=w205, "error in (no error)"=w203, "Section Formatted Cluster"=w202, "refnum"=w204) -> ("error out"=w200:errorcluster, "dup refnum"=w201:T2)  [unwired: 6 in]
              }
              frame True {
              }
            }
          }
        }
      }
    }
    frame "浮标" {
      w293 = enum16{"PLC", "ZLAN", "ART"}[] [enum."ART"] items=["PLC", "ZLAN", "ART"]
      w294 = enum32{"禁用告警", "闭合告警", "断开告警"}[] [enum."闭合告警"] items=["禁用告警", "闭合告警", "断开告警"]
      w295 = T5 [enum."AI1"] items=["AI0", "AI1", "AI2", "AI3", "AI4", "DI0", "DI1", "DI2", "DI3", "DI4", "DI5", "DI6", "DI7", "DO0", "DO1", "DO2", "DO3", "DO4", "DO5", "DO6", "DO7", "X0", "X1", "X2", "X3", "X4", "X5", "X6", "X7", "X8", "X9"]
      n80 = case shown="\"无配置开机恢复\", 默认" w291 {
        tunnel: [w306 TRUE ("empty?")] -> w292
        frame "无配置开机恢复", Default {
          n81 = global read "断电保存全局变量.vi" "配置ItemNames"() -> (w307:string[][])
          n82 = Empty Array?(array=w307) -> (empty?=w306:bool)
        }
        frame "手动恢复" {
        }
      }
      n83 = for {
        tunnel: string[] ["温湿度监测"] -> [w352] mode=indexing
        tunnel: w304 -> [w356]
        tunnel: w303 -> [w355]
        tunnel: w295 -> [w351] mode=indexing
        tunnel: w294 -> [w350] mode=indexing
        tunnel: w293 -> [w349] mode=indexing
        tunnel: [w348] -> w302
        tunnel: [w347] -> w301
        tunnel: w291 -> [w343]
        n84 = call <userlib>:"Read Section Cluster__ogtk.vi"("section (optional)"=w352, "error in (no error)"=w355, "Section Formatted Cluster Type"=T4 {"监测项描述:输出"="烟雾监测", "端口"=enum."X8", "告警方式"=enum."闭合告警", "传感器型号"=enum."PLC"} ("簇1输入"), "refnum"=w356) -> ("error out"=w353:errorcluster, "all found?"=w345:bool, "dup refnum"=w354:T2)  [unwired: 3 in, 2 out]
        n85 = case shown="\"无配置开机恢复\", 默认" w343 {
          tunnel: [w357 FALSE] -> w344
          tunnel: w345 -> [w357 _]
          frame "无配置开机恢复", Default {
          }
          frame "手动恢复" {
          }
        }
        n86 = case shown="假" w344 {
          tunnel: w354 -> [w372 w420]
          tunnel: w353 -> [w371 w419]
          tunnel: w352 -> [w362 _]
          tunnel: w351 -> [w370 _]
          tunnel: w350 -> [w369 _]
          tunnel: w349 -> [w368 _]
          tunnel: [w367 w420] -> w348
          tunnel: [w366 w419] -> w347
          frame False {
            n87 = Bundle By Name(cluster=T1 {"监测项描述:输出"="", "端口"=enum."AI0", "告警方式"=enum."禁用告警", "传感器型号"=enum."PLC", "声光告警启用"=FALSE} ("簇1输入"), "监测项描述:输出"=w362, "端口"=w370, "告警方式"=w369, "传感器型号"=w368, "声光告警启用"=FALSE) -> (w363:T1)
            n88 = global read "断电保存全局变量.vi" "IO监测配置输入"() -> (w365:T6)
            n89 = global read "断电保存全局变量.vi" "监测设备配置"() -> (w361:T7)
            n90 = call <userlib>:"Write Section Cluster__ogtk.vi"("section (optional)"=w362, "error in (no error)"=w371, "Section Formatted Cluster"=w363, "refnum"=w372) -> ("error out"=w366:errorcluster, "dup refnum"=w367:T2)  [unwired: 6 in]
            n91 = case shown="\"温湿度监测\"" w362 {
              tunnel: w365 -> [w374 w378 w382 w388 w394 w400 w406 w412 w418]
              tunnel: [w374 w378 w382 w387 w393 w399 w405 w411 w417] -> w364
              tunnel: w363 -> [_ _ _ w386 w392 w398 w404 w410 w416]
              tunnel: w361 -> [w373 w377 w381 w385 w390 w397 w403 w409 w415]
              tunnel: [w373 w375 w380 w384 w391 w396 w402 w408 w414] -> _
              frame "假", Default {
              }
              frame "市电监测" {
                n92 = Bundle By Name(cluster=w377, "市电监测"=TRUE) -> (w375:T7)
              }
              frame "空调监测" {
                n93 = Bundle By Name(cluster=w381, "空调监测"=TRUE) -> (w380:T7)
              }
              frame "漏水监测" {
                n94 = Bundle By Name(cluster=w388, "漏水监测配置"=w386) -> (w387:T6)
                n95 = Bundle By Name(cluster=w385, "漏水监测"=TRUE) -> (w384:T7)
              }
              frame "门禁开关监测" {
                n96 = Bundle By Name(cluster=w394, "门禁开关监测配置"=w392) -> (w393:T6)
                n97 = Bundle By Name(cluster=w390, "门禁开关监测"=TRUE) -> (w391:T7)
              }
              frame "温湿度监测" {
                n98 = Bundle By Name(cluster=w400, "温湿度监测配置"=w398) -> (w399:T6)
                n99 = Bundle By Name(cluster=w397, "温度湿度"=TRUE) -> (w396:T7)
              }
              frame "烟雾监测" {
                n100 = Bundle By Name(cluster=w406, "烟雾监测配置"=w404) -> (w405:T6)
                n101 = Bundle By Name(cluster=w403, "温度湿度"=TRUE) -> (w402:T7)
              }
              frame "冰箱监测" {
                n102 = Bundle By Name(cluster=w412, "冰箱监测配置"=w410) -> (w411:T6)
                n103 = Bundle By Name(cluster=w409, "冰箱监测"=TRUE ("市电监测")) -> (w408:T7)
              }
              frame "排气扇监测" {
                n104 = Bundle By Name(cluster=w418, "排气扇监测配置"=w416) -> (w417:T6)
                n105 = Bundle By Name(cluster=w415, "排气扇监测"=TRUE) -> (w414:T7)
              }
            }
            n106 = global write "断电保存全局变量.vi" "IO监测配置输入"(w364) -> ()
          }
          frame True {
          }
        }
      }
      n107 = case shown="真" w292 {
        frame False {
        }
        frame True {
          n108 = global write "断电保存全局变量.vi" "配置ItemNames"(string[][] [["1", "温湿度监测", "ART", "IO连接", "端口:AI1 闭合告警 启用声光告警", "编辑", "删除"], ["2", "蓄电池监测", "太阳能控制器-MPPT12", "串口连接", "端口:COM8 站号:1 波特率:115200", "编辑", "删除"]] ("配置ItemNames")) -> ()
        }
      }
      n109 = for {
        tunnel: w302 -> [w322]
        tunnel: w301 -> [w321]
        tunnel: string[] ["蓄电池监测"] -> [w320] mode=indexing
        tunnel: [w317] -> w299
        tunnel: [w316] -> w298
        tunnel: string[] ["COM1"] -> [w315] mode=indexing
        tunnel: string[] ["太阳能控制器-MPPT12"] -> [w314] mode=indexing
        tunnel: w291 -> [w310]
        n110 = call <userlib>:"Read Section Cluster__ogtk.vi"("section (optional)"=w320, "error in (no error)"=w321, "Section Formatted Cluster Type"=T3 {"监测项描述:输出"="", "连接方式"=enum."串口", "端口"="", "IP address:"="", "Port:"="", "站号"=19200, "传感器型号"="", "波特率"=19200, "data bits"=8, "停止位"=10, "奇偶校验"=0} ("输出簇"), "refnum"=w322) -> ("error out"=w318:errorcluster, "all found?"=w312:bool, "dup refnum"=w319:T2)  [unwired: 3 in, 2 out]
        n111 = case shown="\"无配置开机恢复\", 默认" w310 {
          tunnel: [w323 FALSE] -> w311
          tunnel: w312 -> [w323 _]
          frame "无配置开机恢复", Default {
          }
          frame "手动恢复" {
          }
        }
        n112 = case shown="假" w311 {
          tunnel: w320 -> [w339 _]
          tunnel: w319 -> [w338 w342]
          tunnel: w318 -> [w337 w341]
          tunnel: [w335 w342] -> w317
          tunnel: [w334 w341] -> w316
          tunnel: w315 -> [w333 _]
          tunnel: w314 -> [w331 _]
          frame False {
            w325 = "" ("IP address:")
            n113 = Bundle By Name(cluster=T3 {"监测项描述:输出"="", "连接方式"=enum."串口", "端口"="", "IP address:"="", "Port:"="", "站号"=19200, "传感器型号"="", "波特率"=19200, "data bits"=8, "停止位"=10, "奇偶校验"=0} ("输出簇"), "监测项描述:输出"=w339, "端口"=w333, "站号"=u64 1, "传感器型号"=w331, "波特率"=u64 115200, "停止位"=u16 10, "奇偶校验"=u16 0, "data bits"=u64 8, "连接方式"=enum16{"串口", "TCP"}."串口", "IP address:"=w325, "Port:"=w325) -> (w336:T3)
            n114 = call <userlib>:"Write Section Cluster__ogtk.vi"("section (optional)"=w339, "error in (no error)"=w337, "Section Formatted Cluster"=w336, "refnum"=w338) -> ("error out"=w334:errorcluster, "dup refnum"=w335:T2)  [unwired: 6 in]
          }
          frame True {
          }
        }
      }
    }
    frame "浮船" {
      w424 = enum16{"串口", "TCP"}[] [enum."串口", enum."串口", enum."TCP"] items=["串口", "TCP"]
      w427 = enum16{"PLC", "ZLAN", "ART"}[] [enum."ART", enum."ZLAN", enum."ZLAN", enum."ZLAN", enum."ZLAN", enum."ZLAN", enum."ZLAN"] items=["PLC", "ZLAN", "ART"]
      w428 = T5 [enum."AI4", enum."DI0", enum."DI1", enum."DI2", enum."DI4", enum."DI7", enum."DO0"] items=["AI0", "AI1", "AI2", "AI3", "AI4", "DI0", "DI1", "DI2", "DI3", "DI4", "DI5", "DI6", "DI7", "DO0", "DO1", "DO2", "DO3", "DO4", "DO5", "DO6", "DO7", "X0", "X1", "X2", "X3", "X4", "X5", "X6", "X7", "X8", "X9"]
      w429 = enum32{"禁用告警", "闭合告警", "断开告警"}[] [enum."闭合告警", enum."闭合告警", enum."闭合告警", enum."闭合告警", enum."闭合告警", enum."闭合告警", enum."闭合告警"] items=["禁用告警", "闭合告警", "断开告警"]
      n115 = case shown="\"无配置开机恢复\", 默认" w425 {
        tunnel: [w440 TRUE ("empty?")] -> w426
        frame "无配置开机恢复", Default {
          n116 = global read "断电保存全局变量.vi" "配置ItemNames"() -> (w441:string[][])
          n117 = Empty Array?(array=w441) -> (empty?=w440:bool)
        }
        frame "手动恢复" {
        }
      }
      n118 = for {
        tunnel: string[] ["温湿度监测", "漏水监测", "烟雾监测", "门禁开关监测", "门禁开关监测2", "冰箱监测", "排气扇监测"] -> [w491] mode=indexing
        tunnel: w438 -> [w495]
        tunnel: w437 -> [w494]
        tunnel: w428 -> [w490] mode=indexing
        tunnel: w429 -> [w489] mode=indexing
        tunnel: w427 -> [w488] mode=indexing
        tunnel: [w487] -> w436
        tunnel: [w486] -> w435
        tunnel: w425 -> [w484]
        n119 = call <userlib>:"Read Section Cluster__ogtk.vi"("section (optional)"=w491, "error in (no error)"=w494, "Section Formatted Cluster Type"=T4 {"监测项描述:输出"="烟雾监测", "端口"=enum."X8", "告警方式"=enum."闭合告警", "传感器型号"=enum."PLC"} ("簇1输入"), "refnum"=w495) -> ("error out"=w492:errorcluster, "all found?"=w482:bool, "dup refnum"=w493:T2)  [unwired: 3 in, 2 out]
        n120 = case shown="\"无配置开机恢复\", 默认" w484 {
          tunnel: [w496 FALSE] -> w483
          tunnel: w482 -> [w496 _]
          frame "无配置开机恢复", Default {
          }
          frame "手动恢复" {
          }
        }
        n121 = case shown="假" w483 {
          tunnel: w493 -> [w511 w565]
          tunnel: w492 -> [w510 w564]
          tunnel: w491 -> [w501 _]
          tunnel: w490 -> [w509 _]
          tunnel: w489 -> [w508 _]
          tunnel: w488 -> [w507 _]
          tunnel: [w506 w565] -> w487
          tunnel: [w505 w564] -> w486
          frame False {
            n122 = Bundle By Name(cluster=T1 {"监测项描述:输出"="", "端口"=enum."AI0", "告警方式"=enum."禁用告警", "传感器型号"=enum."PLC", "声光告警启用"=FALSE} ("簇1输入"), "监测项描述:输出"=w501, "端口"=w509, "告警方式"=w508, "传感器型号"=w507, "声光告警启用"=FALSE) -> (w502:T1)
            n123 = global read "断电保存全局变量.vi" "IO监测配置输入"() -> (w504:T6)
            n124 = global read "断电保存全局变量.vi" "监测设备配置"() -> (w500:T7)
            n125 = call <userlib>:"Write Section Cluster__ogtk.vi"("section (optional)"=w501, "error in (no error)"=w510, "Section Formatted Cluster"=w502, "refnum"=w511) -> ("error out"=w505:errorcluster, "dup refnum"=w506:T2)  [unwired: 6 in]
            n126 = case shown="\"冰箱监测\"" w501 {
              tunnel: w504 -> [w513 w517 w521 w527 w533 w539 w545 w551 w557 w563]
              tunnel: [w513 w517 w521 w526 w532 w538 w544 w550 w556 w562] -> w503
              tunnel: w502 -> [_ _ _ w525 w531 w537 w543 w549 w555 w561]
              tunnel: w500 -> [w512 w516 w520 w524 w529 w535 w542 w548 w554 w560]
              tunnel: [w512 w514 w519 w523 w530 w536 w541 w547 w553 w559] -> _
              frame "假", Default {
              }
              frame "市电监测" {
                n127 = Bundle By Name(cluster=w516, "市电监测"=TRUE) -> (w514:T7)
              }
              frame "空调监测" {
                n128 = Bundle By Name(cluster=w520, "空调监测"=TRUE) -> (w519:T7)
              }
              frame "漏水监测" {
                n129 = Bundle By Name(cluster=w527, "漏水监测配置"=w525) -> (w526:T6)
                n130 = Bundle By Name(cluster=w524, "漏水监测"=TRUE) -> (w523:T7)
              }
              frame "门禁开关监测" {
                n131 = Bundle By Name(cluster=w533, "门禁开关监测配置"=w531) -> (w532:T6)
                n132 = Bundle By Name(cluster=w529, "门禁开关监测"=TRUE) -> (w530:T7)
              }
              frame "门禁开关监测2" {
                n133 = Bundle By Name(cluster=w539, "门禁开关监测配置2"=w537) -> (w538:T6)
                n134 = Bundle By Name(cluster=w535, "门禁开关监测2"=TRUE ("门禁开关监测")) -> (w536:T7)
              }
              frame "温湿度监测" {
                n135 = Bundle By Name(cluster=w545, "温湿度监测配置"=w543) -> (w544:T6)
                n136 = Bundle By Name(cluster=w542, "温度湿度"=TRUE) -> (w541:T7)
              }
              frame "烟雾监测" {
                n137 = Bundle By Name(cluster=w551, "烟雾监测配置"=w549) -> (w550:T6)
                n138 = Bundle By Name(cluster=w548, "温度湿度"=TRUE) -> (w547:T7)
              }
              frame "冰箱监测" {
                n139 = Bundle By Name(cluster=w557, "冰箱监测配置"=w555) -> (w556:T6)
                n140 = Bundle By Name(cluster=w554, "冰箱监测"=TRUE ("市电监测")) -> (w553:T7)
              }
              frame "排气扇监测" {
                n141 = Bundle By Name(cluster=w563, "排气扇监测配置"=w561) -> (w562:T6)
                n142 = Bundle By Name(cluster=w560, "排气扇监测"=TRUE) -> (w559:T7)
              }
            }
            n143 = global write "断电保存全局变量.vi" "IO监测配置输入"(w503) -> ()
          }
          frame True {
          }
        }
      }
      n144 = case shown="真" w426 {
        frame False {
        }
        frame True {
          n145 = global write "断电保存全局变量.vi" "配置ItemNames"(string[][] [["1", "温湿度监测", "ZLAN", "IO连接", "端口:AI4 闭合告警 启用声光告警", "编辑", "删除"], ["2", "漏水监测", "ZLAN", "IO连接", "端口:DI0 闭合告警 启用声光告警", "编辑", "删除"], ["3", "烟雾监测", "ZLAN", "IO连接", "端口:DI1 闭合告警 启用声光告警", "编辑", "删除"], ["4", "门禁开关监测", "ZLAN", "IO连接", "端口:DI2 断开告警 启用声光告警", "编辑", "删除"], ["5", "门禁开关监测2", "ZLAN", "IO连接", "端口:DI4 启用声光告警", "编辑", "删除"], ["5", "冰箱监测", "ZLAN", "IO连接", "端口:DO2 闭合告警 启用声光告警", "编辑", "删除"], ["6", "排气扇监测", "ZLAN", "IO连接", "端口:DO3 闭合告警 启用声光告警", "编辑", "删除"], ["7", "蓄电池监测", "太阳能控制器-MPPT12", "串口连接", "端口:COM1 站号:1 波特率:115200", "编辑", "删除"], ["8", "蓄电池监测2", "太阳能控制器-MPPT24", "串口连接", "端口:COM1 站号:2 波特率:115200", "编辑", "删除"], ["9", "GPS监测", "GPS", "TCP连接", "IP:192.168.1.1 Port:5001 不启用声光告警", "编辑", "删除"]] ("配置ItemNames")) -> ()
        }
      }
      n146 = for {
        tunnel: w436 -> [w460]
        tunnel: w435 -> [w459]
        tunnel: string[] ["蓄电池监测", "蓄电池监测2", "GPS监测"] -> [w458] mode=indexing
        tunnel: [w455] -> w433
        tunnel: [w454] -> w432
        tunnel: string[] ["COM1", "COM1", ""] -> [w453] mode=indexing
        tunnel: string[] ["太阳能控制器-MPPT12", "太阳能控制器-MPPT24", "GPS"] -> [w452] mode=indexing
        tunnel: w425 -> [w450]
        tunnel: w424 -> [w447] mode=indexing
        tunnel: string[] ["", "", "192.168.1.1"] -> [w446] mode=indexing
        tunnel: string[] ["", "", "5001"] -> [w445] mode=indexing
        tunnel: u64[] [1, 2, 1] -> [w444] mode=indexing
        n147 = call <userlib>:"Read Section Cluster__ogtk.vi"("section (optional)"=w458, "error in (no error)"=w459, "Section Formatted Cluster Type"=T3 {"监测项描述:输出"="", "连接方式"=enum."串口", "端口"="", "IP address:"="", "Port:"="", "站号"=19200, "传感器型号"="", "波特率"=19200, "data bits"=8, "停止位"=10, "奇偶校验"=0} ("输出簇"), "refnum"=w460) -> ("error out"=w456:errorcluster, "all found?"=w449:bool, "dup refnum"=w457:T2)  [unwired: 3 in, 2 out]
        n148 = case shown="\"手动恢复\"" w450 {
          tunnel: [w461 FALSE] -> w448
          tunnel: w449 -> [w461 _]
          frame "无配置开机恢复", Default {
          }
          frame "手动恢复" {
          }
        }
        n149 = case shown="假" w448 {
          tunnel: w458 -> [w478 _]
          tunnel: w457 -> [w477 w481]
          tunnel: w456 -> [w476 w480]
          tunnel: [w474 w481] -> w455
          tunnel: [w473 w480] -> w454
          tunnel: w453 -> [w472 _]
          tunnel: w452 -> [w471 _]
          tunnel: w447 -> [w466 _]
          tunnel: w446 -> [w465 _]
          tunnel: w445 -> [w464 _]
          tunnel: w444 -> [w463 _]
          frame False {
            n150 = Bundle By Name(cluster=T3 {"监测项描述:输出"="", "连接方式"=enum."串口", "端口"="", "IP address:"="", "Port:"="", "站号"=19200, "传感器型号"="", "波特率"=19200, "data bits"=8, "停止位"=10, "奇偶校验"=0} ("输出簇"), "监测项描述:输出"=w478, "端口"=w472, "站号"=w463, "传感器型号"=w471, "波特率"=u64 115200, "停止位"=u16 10, "奇偶校验"=u16 0, "data bits"=u64 8, "连接方式"=w466, "IP address:"=w465, "Port:"=w464) -> (w475:T3)
            n151 = call <userlib>:"Write Section Cluster__ogtk.vi"("section (optional)"=w478, "error in (no error)"=w476, "Section Formatted Cluster"=w475, "refnum"=w477) -> ("error out"=w473:errorcluster, "dup refnum"=w474:T2)  [unwired: 6 in]
          }
          frame True {
          }
        }
      }
    }
  }
  n152 = call <vilib>:"Close Config Data.vi"("error in (no error)"=w8, "refnum"=w9) -> ("error out"=w2:errorcluster)  [unwired: 8 in, 1 out]
  n153 = call "save.vi"("error in (no error)"=w2) -> ("error out"=→"error out":errorcluster)  [unwired: 10 in]
